vi "Server Generate Answer Event.vi"(8 "error in":errorcluster, 10 "event data":string, 11 "server event ref":refnum<vi>) -> (0 "error out":errorcluster)   [LabVIEW 2013]
doc: "Sends answer event to server."
uses:
  <vilib>/event_ctls.llb/usereventprio.ctl
  Server Event Answer Ref.ctl
  Server Session.ctl
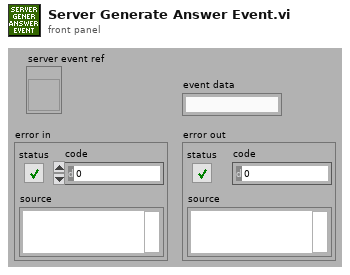
[diagram p1: front panel]
types:
  T1 = typedef "Server Session.ctl" = cluster{"cmd event":variant, "answer event":variant}
  T2 = typedef "Server Event Answer Ref.ctl" = refnum<user-event>
  T3 = typedef "usereventprio.ctl" = enum32{"high priority", "normal priority"}
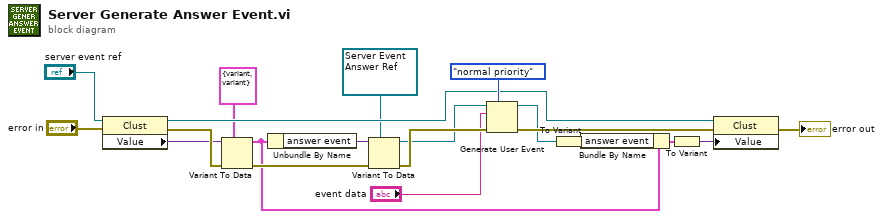
[diagram p0: block diagram]
diagram:
  n1 = property class="Clust"(reference="server event ref", error in="error in") -> (reference out=w17:refnum<vi>, error out=w10:errorcluster, "Value"=w9:variant)
  n2 = Variant To Data(error in=w10, type=T1 {"cmd event"=variant(refnum<user-event> refnum), "answer event"=variant(refnum<user-event> refnum)} ("server"), Variant=w9) -> (data=w4:T1, error out=w8:errorcluster)
  n3 = Unbundle By Name(w4) -> ("answer event"=w6:variant)
  n4 = Variant To Data(error in=w8, type=T2 refnum ("user event out"), Variant=w6) -> (data=w13:T2, error out=w14:errorcluster)
  n5 = Generate User Event(priority (normal)=usereventprio."normal priority", user event=w13, event data cluster="event data", error in=w14) -> (user event out=w16:T2, error out=w19:errorcluster)
  n6 = To Variant(anything=w16) -> (Variant=w3:variant)
  n7 = Bundle By Name(cluster=w4, "answer event"=w3) -> (w5:T1)
  n8 = To Variant(anything=w5) -> (Variant=w2:variant)
  n9 = property class="Clust"(reference=w17, error in=w19, "Value"=w2) -> (error out=→"error out":errorcluster)  [unwired: 1 out]
